vi "Find Added Sections.vi"(9 "Offset":u32, 10 "Reference":string, 11 "Target":string) -> (3 "Sections in Target":T1(array[cluster]))   [LabVIEW 2020]
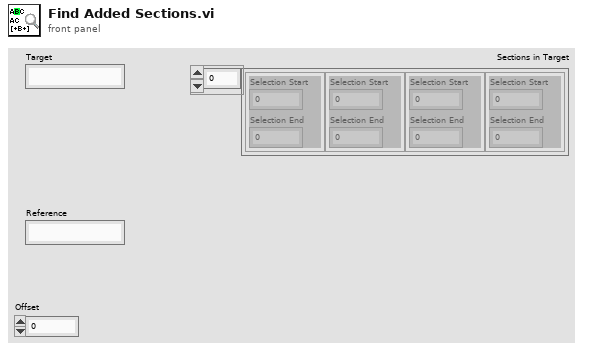
[diagram p1: front panel]
types:
  T1 = cluster{"Selection Start":u32, "Selection End":u32}[]
  T2 = cluster{"Selection Start":u32, "Selection End":u32}
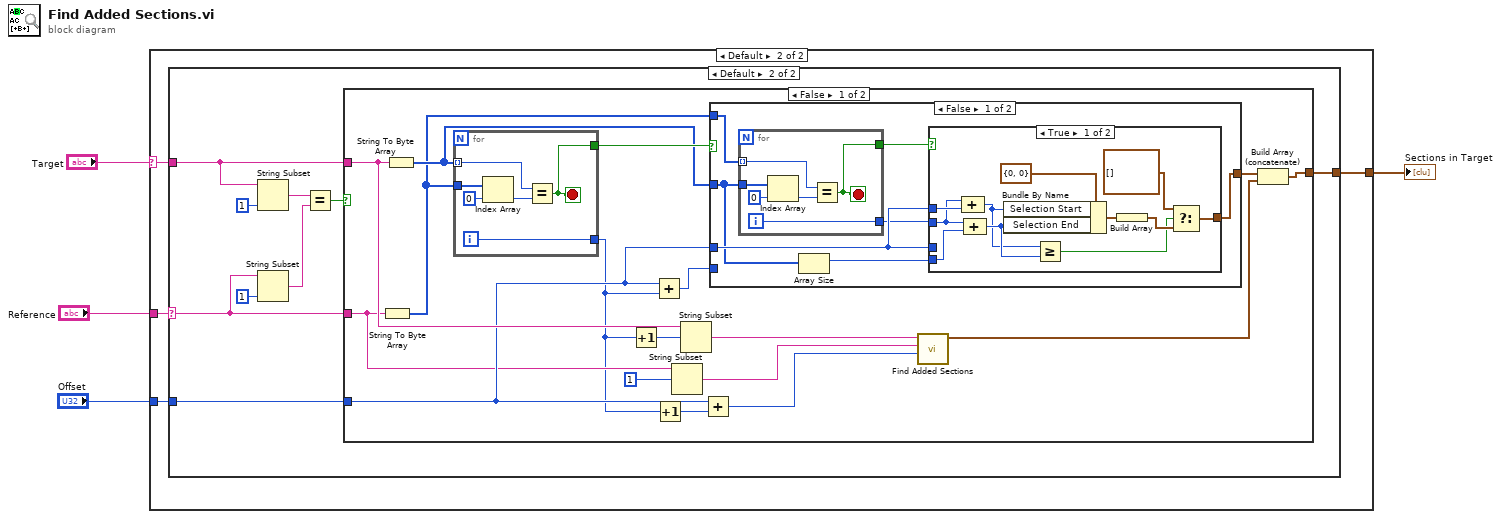
[diagram p0: block diagram]
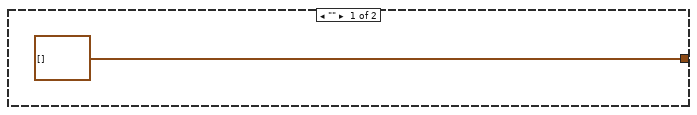
[diagram p2: hidden frame]
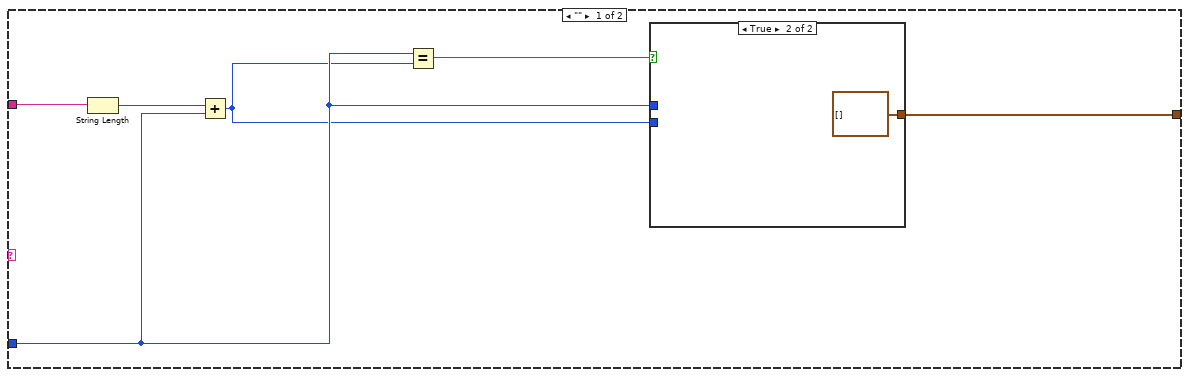
[diagram p3: hidden frame]
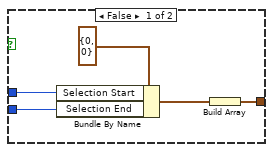
[diagram p4: hidden frame]
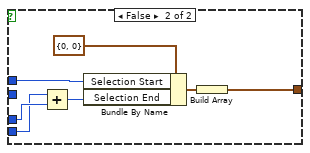
[diagram p5: hidden frame]
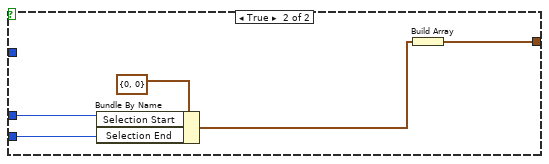
[diagram p6: hidden frame]
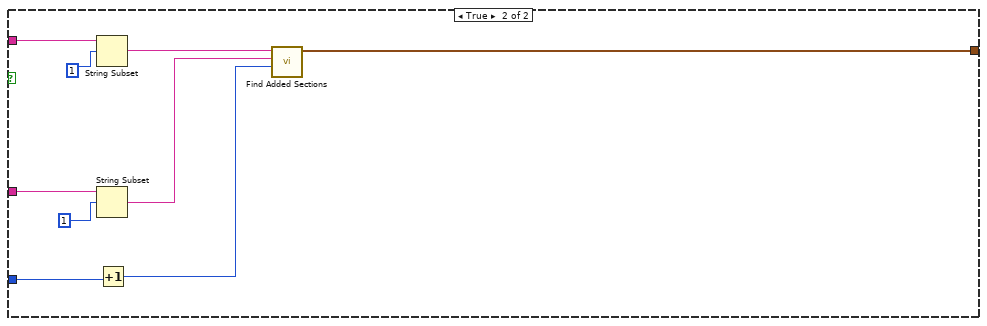
[diagram p7: hidden frame]
diagram:
  n1 = case shown="Default" "Target" {
    selector: "Target" -> [_ w9]
    tunnel: "Reference" -> [_ w8]
    tunnel: [T1 [] w7] -> w2
    tunnel: "Offset" -> [_ w6]
    frame "" {
    }
    frame Default {
      n2 = case shown="Default" w8 {
        selector: w8 -> [_ w24]
        tunnel: w9 -> [w14 w25]
        tunnel: [w15 w23] -> w7
        tunnel: w6 -> [w12 w22]
        frame "" {
          n3 = String Length(string=w14) -> (length=w13:i32)
          n4 = Add(x=w13, y=w12) -> (x+y=w11:u32)
          n5 = Equal?(x=w12, y=w11) -> (x = y?=w10:bool)
          n6 = case shown="True" w10 {
            tunnel: [w18 T1 []] -> w15
            tunnel: w12 -> [w17 _]
            tunnel: w11 -> [w16 _]
            frame False {
              n7 = Bundle By Name(cluster=T2 {"Selection Start"=0, "Selection End"=0} ("Missmatches"), "Selection Start"=w17, "Selection End"=w16) -> (w19:T2)
              n8 = Build Array(w19) -> (w18:T1)
            }
            frame True {
            }
          }
        }
        frame Default {
          n9 = String Subset(string=w25, length (rest)=1 ("length (rest)")) -> (substring=w28:string)  [unwired: 1 in]
          n10 = String Subset(string=w24, length (rest)=1 ("length (rest)")) -> (substring=w27:string)  [unwired: 1 in]
          n11 = Equal?(x=w28, y=w27) -> (x = y?=w26:bool)
          n12 = case shown="False" w26 {
            tunnel: w25 -> [w43 w97]
            tunnel: w24 -> [w40 w96]
            tunnel: [w45 w92] -> w23
            tunnel: w22 -> [w41 w91]
            frame False {
              n13 = String To Byte Array(string=w40) -> (unsigned byte array=w34:u8[])
              n14 = String To Byte Array(string=w43) -> (unsigned byte array=w35:u8[])
              n15 = for {
                tunnel: [w88] -> w32
                tunnel: w35 -> [w86] mode=indexing
                tunnel: w34 -> [w89]
                tunnel: [w85] -> w36
                i -> [w88]
                stop <- w85 stop-if-true
                n16 = Index Array(array=w89, index=0) -> (element=w87:u8)
                n17 = Equal?(x=w86, y=w87) -> (x = y?=w85:bool)
              }
              n18 = Increment(x=w32) -> (x+1=w31:i32)
              n19 = Add(x=w41, y=w32) -> (x+y=w47:u32)
              n20 = Increment(x=w32) -> (x+1=w33:i32)
              n21 = String Subset(string=w40, offset (0)=1) -> (substring=w38:string)  [unwired: 1 in]
              n22 = String Subset(string=w43, offset (0)=w31) -> (substring=w42:string)  [unwired: 1 in]
              n23 = Add(x=w41, y=w33) -> (x+y=w37:u32)
              n24 = case shown="False" w36 {
                tunnel: w47 -> [_ w82]
                tunnel: [w53 w80] -> w46
                tunnel: w41 -> [w51 w81]
                tunnel: w34 -> [w54 _]
                tunnel: w35 -> [w50 _]
                frame False {
                  n25 = for {
                    tunnel: w54 -> [w77] mode=indexing
                    tunnel: w50 -> [w74]
                    tunnel: [w76] -> w52
                    tunnel: [w73] -> w49
                    i -> [w73]
                    stop <- w76 stop-if-true
                    n26 = Index Array(array=w74, index=0) -> (element=w78:u8)
                    n27 = Equal?(x=w77, y=w78) -> (x = y?=w76:bool)
                  }
                  n28 = Array Size(array=w50) -> (size(s)=w48:i32)
                  n29 = case shown="True" w52 {
                    tunnel: w51 -> [_ w68]
                    tunnel: [w61 w70] -> w53
                    tunnel: w51 -> [w60 w69]
                    tunnel: w49 -> [w55 _]
                    tunnel: w48 -> [w62 w66]
                    frame True {
                      n30 = Compound Arithmetic op=ADD(w55, w60) -> (w56:u32)
                      n31 = Compound Arithmetic op=ADD(w55, w62) -> (w59:i32)
                      n32 = Bundle By Name(cluster=T2 {"Selection Start"=0, "Selection End"=0} ("Missmatches"), "Selection Start"=w56, "Selection End"=w59) -> (w64:T2)
                      n33 = Greater Or Equal?(x=w56, y=w59) -> (x >= y?=w58:bool)
                      n34 = Build Array(w64) -> (w63:T1)
                      n35 = Select(t=T1 [] ("f"), s=w58, f=w63) -> (s? t:f=w61:T1)
                    }
                    frame False {
                      n36 = Add(x=w66, y=w68) -> (x+y=w67:u32)
                      n37 = Bundle By Name(cluster=T2 {"Selection Start"=0, "Selection End"=0} ("Missmatches"), "Selection Start"=w69, "Selection End"=w67) -> (w71:T2)
                      n38 = Build Array(w71) -> (w70:T1)
                    }
                  }
                }
                frame True {
                  n39 = Bundle By Name(cluster=T2 {"Selection Start"=0, "Selection End"=0} ("Missmatches"), "Selection Start"=w81, "Selection End"=w82) -> (w79:T2)
                  n40 = Build Array(w79) -> (w80:T1)
                }
              }
              n41 = call "Find Added Sections.vi"("Offset"=w37, "Reference"=w38, "Target"=w42) -> ("Sections in Target"=w44:T1)  [unwired: 8 in]
              n42 = Build Array (concatenate)(w46, w44) -> (w45:T1)
            }
            frame True {
              n43 = String Subset(string=w97, offset (0)=1 ("length (rest)")) -> (substring=w94:string)  [unwired: 1 in]
              n44 = String Subset(string=w96, offset (0)=1 ("length (rest)")) -> (substring=w93:string)  [unwired: 1 in]
              n45 = Increment(x=w91) -> (x+1=w90:u32)
              n46 = call "Find Added Sections.vi"("Offset"=w90, "Reference"=w93, "Target"=w94) -> ("Sections in Target"=w92:T1)  [unwired: 8 in]
            }
          }
        }
      }
    }
  }
  "Sections in Target" <- w2
